vi "ExperimentLogGlobal.vi"() -> ()   [LabVIEW 2020]
panel:
  in  "#Loads&shots":u32
  in  "Experiments Log FileName":string
  in  "Experiments LogName":string
  in  "Experiments Log#":u32
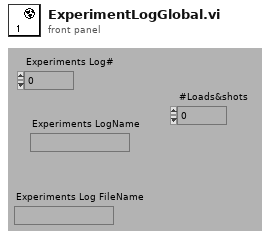
[diagram p1: front panel]
diagram:
